vi "CRYDigital IO Update.vi"(7 "No.VI":i32, 9 "Pattern":T1, 10 "Line selected":T2, 11 "Bits Cluster":T3(array[cluster])) -> (3 "Pattern Out":T1)   [LabVIEW 2013]
uses:
  Typedef Control/CRYResult Cluster Array.ctl
  Typedef Control/CRYResult Cluster.ctl
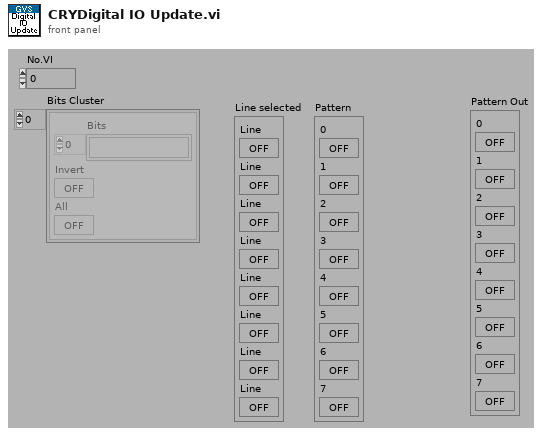
[diagram p1: front panel]
types:
  T1 = cluster{"0":bool, "1":bool, "2":bool, "3":bool, "4":bool, "5":bool, "6":bool, "7":bool}
  T2 = cluster{"Line":bool, "Line":bool, "Line":bool, "Line":bool, "Line":bool, "Line":bool, "Line":bool, "Line":bool}
  T3 = cluster{"Bits":string[], "Invert":bool, "All":bool}[]
  T4 = typedef "CRYResult Cluster Array.ctl" = T5[]
  T5 = typedef "CRYResult Cluster.ctl" = cluster{"Name":string, "Margin":dbl, "unit":string, "Verdict":bool, "Limit":string, "Max/Min":string, "protected":bool, "Step No.":i32, "Test Info":string, "AutoProtect":bool}
  T6 = cluster{"[0]":bool, "[1]":bool, "[2]":bool, "[3]":bool, "[4]":bool, "[5]":bool, "[6]":bool, "[7]":bool}
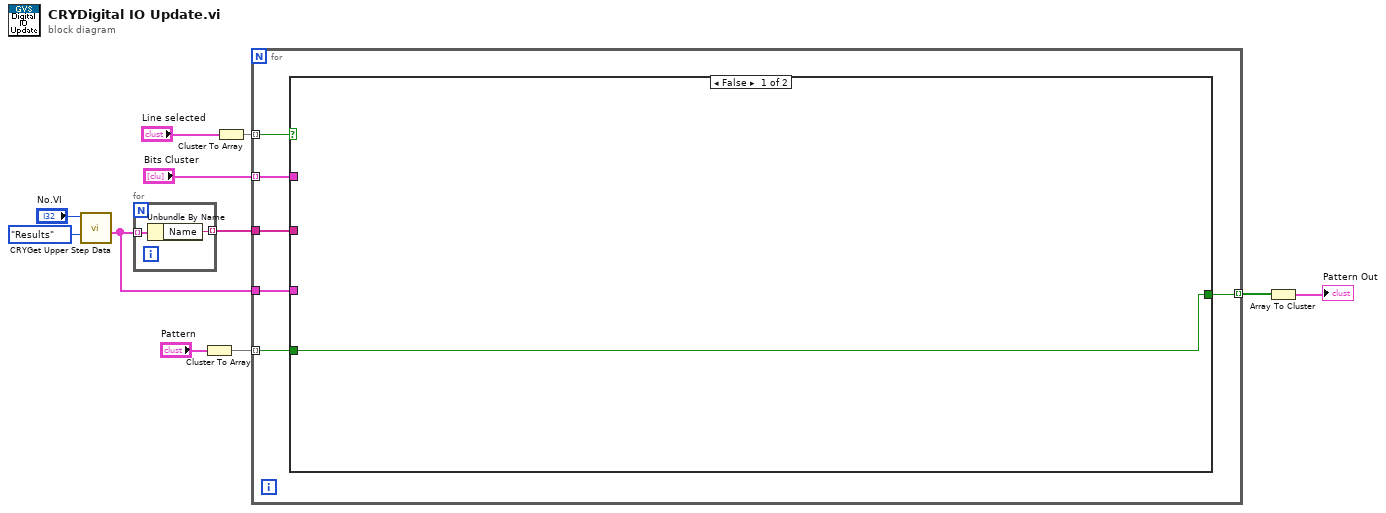
[diagram p0: block diagram]
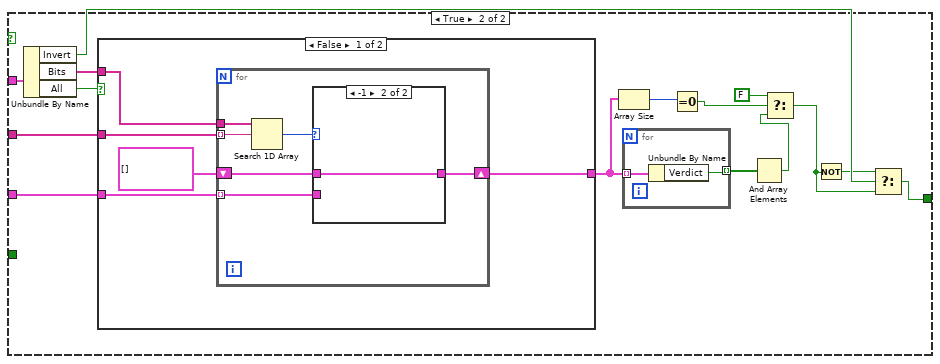
[diagram p2: hidden frame]
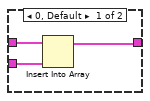
[diagram p3: hidden frame]
diagram:
  n1 = call "CRYGet Upper Step Data.vi"("Type In"=enum16{"Curves", "Values", "Results", "WFM"}."Results", "No.VI"="No.VI") -> ("Result array"=w1:T4)  [unwired: 9 out]
  n2 = for {
    tunnel: w1 -> [w13] mode=indexing
    tunnel: [w12] -> w2 mode=indexing
    n3 = Unbundle By Name(w13) -> ("Name"=w12:string)
  }
  n4 = Cluster To Array(cluster="Pattern") -> (array=w10:bool[])
  n5 = Cluster To Array(cluster="Line selected") -> (array=w11:bool[])
  n6 = for {
    tunnel: "Bits Cluster" -> [w19] mode=indexing
    tunnel: w2 -> [w18]
    tunnel: w11 -> [w17] mode=indexing
    tunnel: [w16] -> w9 mode=indexing
    tunnel: w10 -> [w15] mode=indexing
    tunnel: w1 -> [w14]
    n7 = case shown="False" w17 {
      tunnel: w19 -> [_ w35]
      tunnel: w18 -> [_ w34]
      tunnel: [w20 w28] -> w16
      tunnel: w15 -> [w20 _]
      tunnel: w14 -> [_ w32]
      frame False {
      }
      frame True {
        n8 = Unbundle By Name(w35) -> ("Invert"=w29:bool, "Bits"=w30:string[], "All"=w33:bool)
        n9 = case shown="False" w33 {
          tunnel: w34 -> [w41 _]
          tunnel: w30 -> [w42 _]
          tunnel: w32 -> [w38 w53]
          tunnel: [w39 w53] -> w26
          frame False {
            n10 = for {
              tunnel: w41 -> [w44] mode=indexing
              tunnel: w42 -> [w45]
              shift-right: [w46] -> w39
              shift-left: T4 [] ("Result array") -> [w47]
              tunnel: w38 -> [w43] mode=indexing
              n11 = Search 1D Array(1D array=w45, element=w44) -> (index of element=w48:i32)  [unwired: 1 in]
              n12 = case shown="-1" w48 {
                tunnel: w47 -> [w51 w52]
                tunnel: [w50 w52] -> w46
                tunnel: w43 -> [w49 _]
                frame 0, Default {
                  n13 = Insert Into Array(array=w51, new element=w49) -> (w50:T4)  [unwired: 1 in]
                }
                frame -1 {
                }
              }
            }
          }
          frame True {
          }
        }
        n14 = Array Size(array=w26) -> (size(s)=w25:i32)
        n15 = for {
          tunnel: w26 -> [w37] mode=indexing
          tunnel: [w36] -> w31 mode=indexing
          n16 = Unbundle By Name(w37) -> ("Verdict"=w36:bool)
        }
        n17 = Equal To 0?(x=w25) -> (x = 0?=w24:bool)
        n18 = And Array Elements(Boolean array=w31) -> (logical AND=w22:bool)
        n19 = Select(t=FALSE, s=w24, f=w22) -> (s? t:f=w23:bool)
        n20 = Not(x=w23) -> (.not. x?=w27:bool)
        n21 = Select(t=w27, s=w29, f=w23) -> (s? t:f=w28:bool)
      }
    }
  }
  n22 = Array To Cluster(array=w9) -> (cluster=→"Pattern Out":T6)
